vi "RichToFlatcif_channelcore_GetChannelsRequest.vi"(5 "OutputClusterType":T1, 11 "InputCluster":T2) -> (3 "OutputCluster":T1)   [LabVIEW 2021, in "CIFCoreChannel_client.lvlib"]
uses:
  CIFCoreChannel_client.lvlib
  cif_channelcore_GetChannelsRequest.ctl
  cif_channelcore_GetChannelsRequest_Flat.ctl
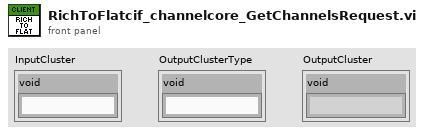
[diagram p1: front panel]
types:
  T1 = typedef "CIFCoreChannel_client.lvlib/cif_channelcore_GetChannelsRequest_Flat.ctl" = cluster{"void":string}
  T2 = typedef "CIFCoreChannel_client.lvlib/cif_channelcore_GetChannelsRequest.ctl" = cluster{"void":string}
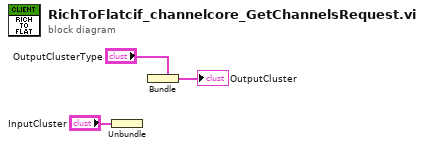
[diagram p0: block diagram]
diagram:
  n1 = Unbundle "Unbundle"("InputCluster") -> ()  [unwired: 1 out]
  n2 = Bundle "Bundle"(cluster="OutputClusterType") -> (→"OutputCluster":T1)  [unwired: 1 in]
